vi "Disable Source Separation (Library).vi"(8 "Error In":errorcluster, 11 "Library":refnum<vi>) -> (0 "Error Out":errorcluster, 3 "Modded Library":refnum<vi>)   [LabVIEW 2014]
doc: "Copyright (c) 2018 Sze Howe Koh\n\nThis Source Code Form is subject to the terms of the Mozilla Public License, v. 2.0. If a copy of the MPL was not distributed with this file, You can obtain one at http://mozilla.org/MPL/2.0/."
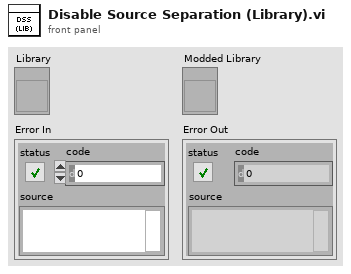
[diagram p1: front panel]
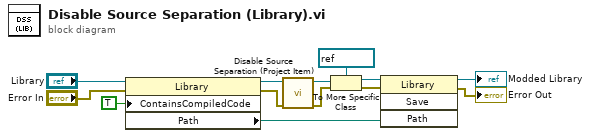
[diagram p0: block diagram]
diagram:
  n1 = property class="Library"(reference="Library", error in="Error In", "ContainsCompiledCode"=TRUE ("Contains Compiled Code")) -> (reference out=w12:refnum<vi>, error out=w3:errorcluster, "Path"=w8:path)
  n2 = call "Disable Source Separation (Project Item).vi"("Error In"=w3, "Project Item"=w12) -> ("Error Out"=w4:errorcluster, "Project Item Dup"=w11:refnum<vi>)  [unwired: 8 in]
  n3 = To More Specific Class(target class=refnum<vi> refnum ("Library"), reference=w11, error in=w4) -> (specific class reference=w9:refnum<vi>, error out=w6:errorcluster)
  n4 = invoke class="Library" method="Save"(reference=w9, error in=w6, "Path"=w8) -> (reference out=→"Modded Library":refnum<vi>, error out=→"Error Out":errorcluster)  [unwired: 1 in, 2 out]
